vi "Peak Detection.vi"() -> ()   [LabVIEW 2015]
uses:
  <vilib>/Utility/file.llb/Read Delimited Spreadsheet (DBL).vi
  <userlib>/_OpenG.lib/array/array.llb/Sort 2D Array (DBL)__ogtk.vi
  <vilib>/Analysis/NI_AALPro.lvlib
  <vilib>/Analysis/NI_AAL_SigProc.lvlib
panel:
  out "Within 5 Peaks of each other?":bool[](array[boolean])
  out "Smoothed Data":dbl[](array[numeric])
  out "isDecreasing":bool[](array[boolean])
  out "isIncreasing":bool[](array[boolean])
  out "(2nd) Zero Crossing Amplitude and Index":dbl[][](array[numeric])
  out "(1st) Zero Crossing Amplitude and Index":dbl[][](array[numeric])
  out "Sorted 2D Array":sgl[][](array[numeric])
  in  "MinumumPeakHeightThresholdCounts":dbl format="%#_13g"
  out "?":cluster{dbl, dbl}[](graph)=[{0.0, 0.0}, {0.0, 0.0}, {366.0, 183.0}, {15.0, 190.5}, {11.0, 13.0}, {18.0, 14.5}, {9.0, 13.5}, {8.0, 8.5}, {0.0, 4.0}, {3.0, 1.5}, {11.0, 7.0}, {12.0, 11.5}, {16.0, 14.0}, {22.0, 19.0}, {16.0, 19.0}, {26.0, 21.0}, {17.0, 21.5}, {11.0, 14.0}, {1.0, 6.0}, {1.0, 1.0}, {0.0, 0.5}, {3.0, 1.5}, {4.0, 3.5}, {6.0, 5.0}, {16.0, 11.0}, {25.0, 20.5}, {53.0, 39.0}, {91.0, 72.0}, {204.0, 147.5}, {638.0, 421.0}, {2954.0, 1796.0}, {4799.0, 3876.5}, {6341.0, 5570.0}, {6306.0, 6323.5}, {6336.0, 6321.0}, {5904.0, 6120.0}, {5304.0, 5604.0}, {2436.0, 3870.0}, {107.0, 1271.5}, {17.0, 62.0}, {23.0, 20.0}, {82.0, 52.5}, {127.0, 104.5}, {93.0, 110.0}, {124.0, 108.5}, {109.0, 116.5}, {89.0, 99.0}, {58.0, 73.5}, {2.0, 30.0}, {3.0, 2.5}, {14.0, 8.5}, {25.0, 19.5}, {32.0, 28.5}, {37.0, 34.5}, {36.0, 36.5}, {29.0, 32.5}, {22.0, 25.5}, {9.0, 15.5}, {2.0, 5.5}, {1.0, 1.5}, {3.0, 2.0}, {5.0, 4.0}, {2.0, 3.5}, {2.0, 2.0}, {10.0, 6.0}, {14.0, 12.0}, {21.0, 17.5}, {22.0, 21.5}, {14.0, 18.0}, {24.0, 19.0}, {17.0, 20.5}, {10.0, 13.5}, {7.0, 8.5}, {10.0, 8.5}, {20.0, 15.0}, {36.0, 28.0}, {22.0, 29.0}, {56.0, 39.0}, {43.0, 49.5}, {64.0, 53.5}, {49.0, 56.5}, {23.0, 36.0}, {5.0, 14.0}, {11.0, 8.0}, {8.0, 9.5}, {17.0, 12.5}, {24.0, 20.5}, {20.0, 22.0}, {19.0, 19.5}, {28.0, 23.5}, {13.0, 20.5}, {14.0, 13.5}, {28.0, 21.0}, {61.0, 44.5}, {115.0, 88.0}, {186.0, 150.5}, {306.0, 246.0}, {305.0, 305.5}, {294.0, 299.5}, {338.0, 316.0}, {235.0, 286.5}, {236.0, 235.5}, {131.0, 183.5}, {51.0, 91.0}, {48.0, 49.5}, {81.0, 64.5}, {87.0, 84.0}, {112.0, 99.5}, {94.0, 103.0}, {103.0, 98.5}, {93.0, 98.0}, {71.0, 82.0}, {39.0, 55.0}, {24.0, 31.5}, {31.0, 27.5}, {51.0, 41.0}, {51.0, 51.0}, {62.0, 56.5}, {58.0, 60.0}, {53.0, 55.5}, {52.0, 52.5}, {62.0, 57.0}, {27.0, 44.5}, {5.0, 16.0}, {8.0, 6.5}, {4.0, 6.0}, {3.0, 3.5}, {3.0, 3.0}, {4.0, 3.5}, {15.0, 9.5}, {8.0, 11.5}, {15.0, 11.5}, {18.0, 16.5}, {15.0, 16.5}, {9.0, 12.0}, {4.0, 6.5}, {2.0, 3.0}, {2.0, 2.0}, {5.0, 3.5}, {7.0, 6.0}, {18.0, 12.5}, {14.0, 16.0}, {8.0, 11.0}, {13.0, 10.5}, {15.0, 14.0}, {40.0, 27.5}, {102.0, 71.0}, {227.0, 164.5}, {319.0, 273.0}, {462.0, 390.5}, {638.0, 550.0}, {643.0, 640.5}, {632.0, 637.5}, {620.0, 626.0}, {481.0, 550.5}, {361.0, 421.0}, {138.0, 249.5}, {121.0, 129.5}, {172.0, 146.5}, {275.0, 223.5}, {272.0, 273.5}, {352.0, 312.0}, {353.0, 352.5}, {267.0, 310.0}, {243.0, 255.0}, {167.0, 205.0}, {66.0, 116.5}, {56.0, 61.0}, {70.0, 63.0}, {93.0, 81.5}, {119.0, 106.0}, {129.0, 124.0}, {117.0, 123.0}, {92.0, 104.5}, {81.0, 86.5}, {48.0, 64.5}, {28.0, 38.0}, {22.0, 25.0}, {17.0, 19.5}, {25.0, 21.0}, {29.0, 27.0}, {34.0, 31.5}, {33.0, 33.5}, {31.0, 32.0}, {26.0, 28.5}, {16.0, 21.0}, {0.0, 8.0}, {0.0, 0.0}, {0.0, 0.0}, {0.0, 0.0}, {0.0, 0.0}, {0.0, 0.0}, {1.0, 0.5}, {2.0, 1.5}, {2.0, 2.0}, {2.0, 2.0}, {2.0, 2.0}, {0.0, 1.0}, {0.0, 0.0}, {3.0, 1.5}, {1.0, 2.0}, {1.0, 1.0}, {0.0, 0.5}, {2.0, 1.0}, {0.0, 1.0}, {0.0, 0.0}, {1.0, 0.5}, {2.0, 1.5}, {6.0, 4.0}, {21.0, 13.5}, {22.0, 21.5}, {33.0, 27.5}, {26.0, 29.5}, {35.0, 30.5}, {38.0, 36.5}, {49.0, 43.5}, {39.0, 44.0}, {23.0, 31.0}, {15.0, 19.0}, {8.0, 11.5}, {18.0, 13.0}, {26.0, 22.0}, {21.0, 23.5}, {37.0, 29.0}, {27.0, 32.0}, {32.0, 29.5}, {27.0, 29.5}, {24.0, 25.5}, {10.0, 17.0}, {6.0, 8.0}, {10.0, 8.0}, {11.0, 10.5}, {15.0, 13.0}, {14.0, 14.5}, {13.0, 13.5}, {10.0, 11.5}, {11.0, 10.5}, {5.0, 8.0}, {2.0, 3.5}, {4.0, 3.0}, {1.0, 2.5}, {5.0, 3.0}, {3.0, 4.0}, {4.0, 3.5}, {4.0, 4.0}, {3.0, 3.5}, {3.0, 3.0}, {2.0, 2.5}, {0.0, 1.0}, {0.0, 0.0}, {0.0, 0.0}, {1.0, 0.5}, {2.0, 1.5}, {1.0, 1.5}, {1.0, 1.0}, {0.0, 0.5}, {0.0, 0.0}, {0.0, 0.0}, {0.0, 0.0}, {0.0, 0.0}, {0.0, 0.0}, {0.0, 0.0}, {1.0, 0.5}, {0.0, 0.5}, {0.0, 0.0}, {0.0, 0.0}, {0.0, 0.0}, {1.0, 0.5}, {0.0, 0.5}, {0.0, 0.0}, {3.0, 1.5}, {2.0, 2.5}, {8.0, 5.0}, {11.0, 9.5}, {9.0, 10.0}, {21.0, 15.0}, {21.0, 21.0}, {11.0, 16.0}, {8.0, 9.5}, {4.0, 6.0}, {2.0, 3.0}, {4.0, 3.0}, {9.0, 6.5}, {12.0, 10.5}, {8.0, 10.0}, {9.0, 8.5}, {11.0, 10.0}, {12.0, 11.5}, {4.0, 8.0}, {5.0, 4.5}, {0.0, 2.5}, {3.0, 1.5}, {7.0, 5.0}, {6.0, 6.5}, {6.0, 6.0}, {4.0, 5.0}, {6.0, 5.0}, {2.0, 4.0}, {1.0, 1.5}, {0.0, 0.5}, {0.0, 0.0}, {1.0, 0.5}, {2.0, 1.5}, {1.0, 1.5}, {1.0, 1.0}, {2.0, 1.5}, {5.0, 3.5}, {1.0, 3.0}, {0.0, 0.5}, {0.0, 0.0}, {0.0, 0.0}, {0.0, 0.0}, {0.0, 0.0}, {0.0, 0.0}, {1.0, 0.5}, {0.0, 0.5}, {0.0, 0.0}, {0.0, 0.0}, {0.0, 0.0}, {0.0, 0.0}, {1.0, 0.5}, {0.0, 0.5}, {0.0, 0.0}, {0.0, 0.0}, {1.0, 0.5}, {0.0, 0.5}, {0.0, 0.0}, {0.0, 0.0}, {0.0, 0.0}, {0.0, 0.0}, {0.0, 0.0}, {0.0, 0.0}, {0.0, 0.0}, {1.0, 0.5}, {2.0, 1.5}, {2.0, 2.0}, {3.0, 2.5}, {2.0, 2.5}, {4.0, 3.0}, {4.0, 4.0}, {3.0, 3.5}, {1.0, 2.0}, {1.0, 1.0}, {3.0, 2.0}, {1.0, 2.0}, {0.0, 0.5}, {2.0, 1.0}, {2.0, 2.0}, {0.0, 1.0}, {1.0, 0.5}, {1.0, 1.0}, {0.0, 0.5}, {1.0, 0.5}, {1.0, 1.0}, {0.0, 0.5}, {0.0, 0.0}, {0.0, 0.0}, {0.0, 0.0}, {1.0, 0.5}, {1.0, 1.0}, {0.0, 0.5}, {0.0, 0.0}, {0.0, 0.0}, {1.0, 0.5}, {0.0, 0.5}, {0.0, 0.0}, {0.0, 0.0}, {2.0, 1.0}, {0.0, 1.0}, {0.0, 0.0}]
  in  "MinimumPeakHeightThresholdFunction":dbl format="%#_13g"
  in  "MinimumPeakWidth":dbl format="%#_13g"
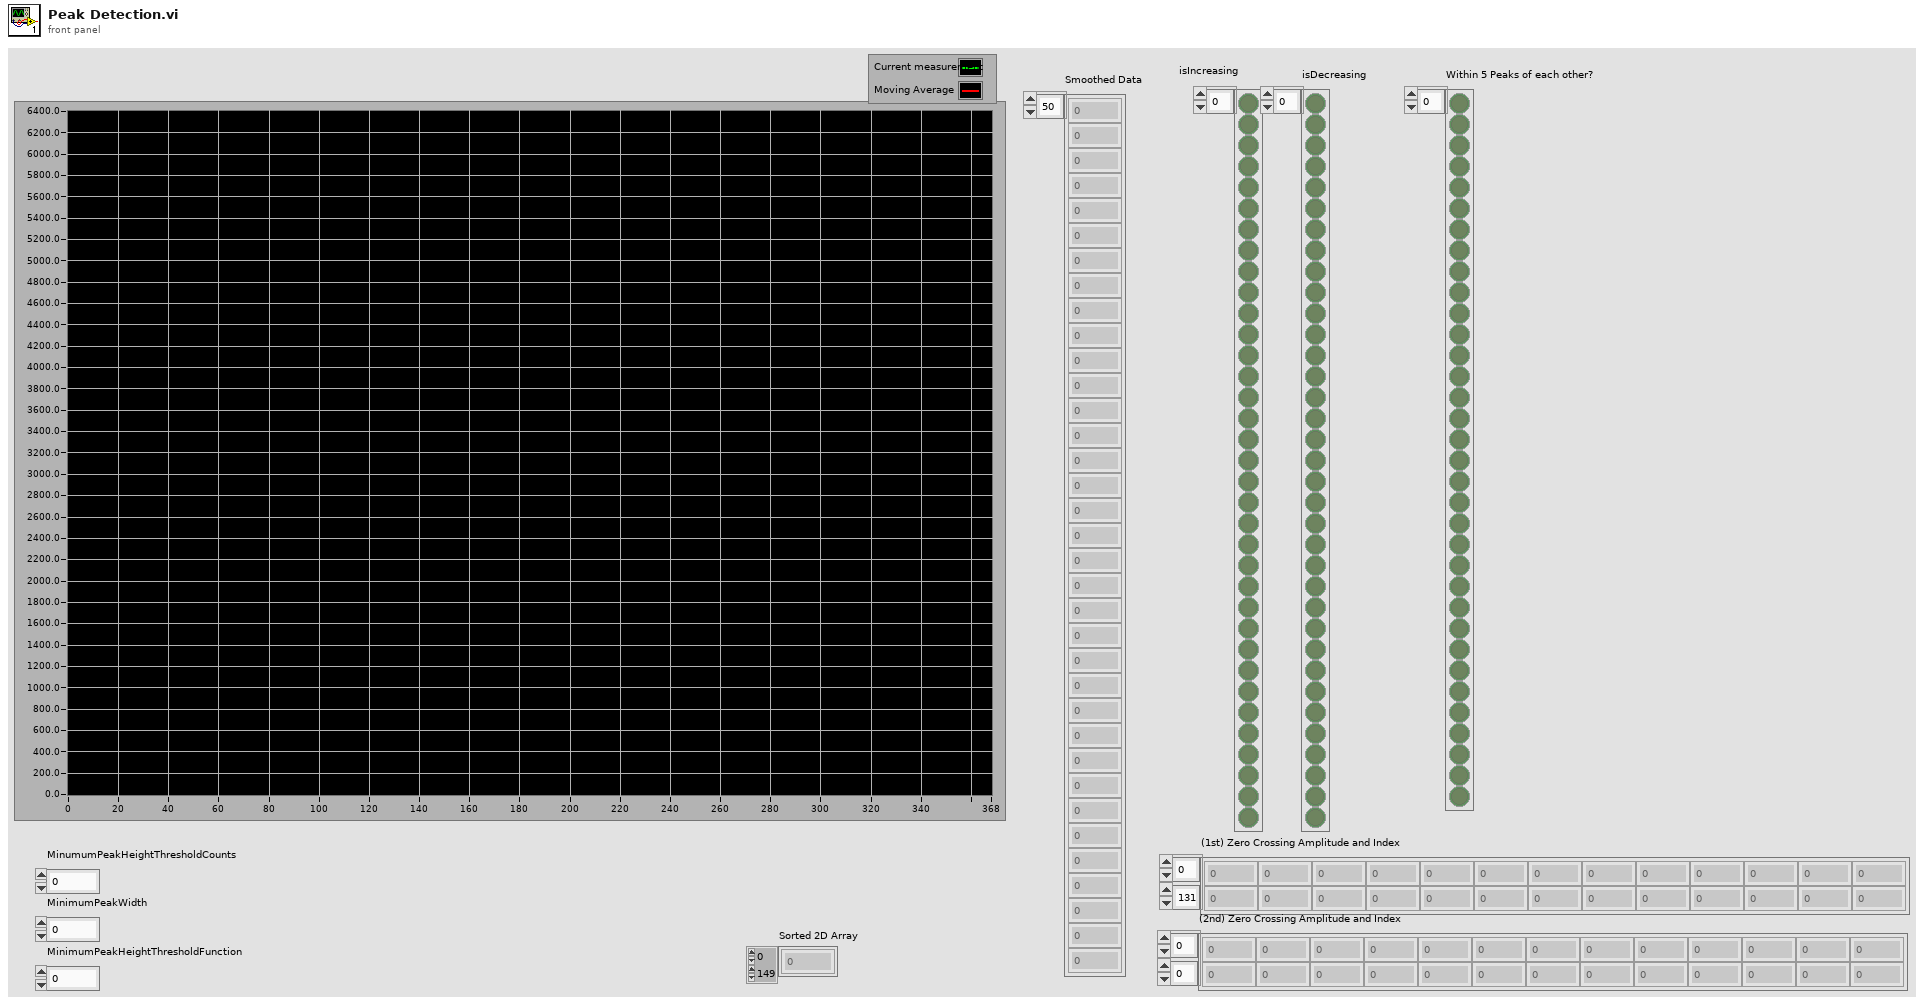
[diagram p1: front panel]
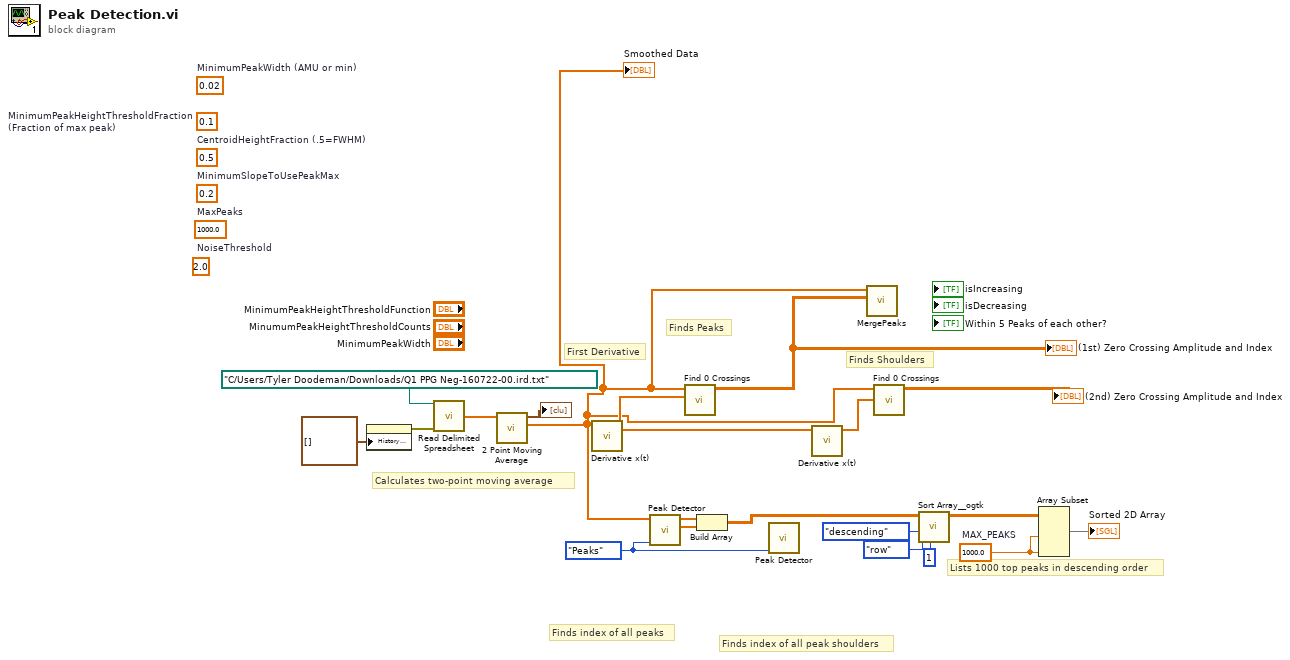
[diagram p0: block diagram]
diagram:
  (unwired) 1000.0  # MaxPeaks
  (unwired) 2.0  # NoiseThreshold
  (unwired) 0.2  # MinimumSlopeToUsePeakMax
  (unwired) 0.5  # CentroidHeightFraction (.5=FWHM)
  (unwired) 0.1  # MinimumPeakHeightThresholdFraction (Fraction of max peak)
  (unwired) 0.02  # MinimumPeakWidth (AMU or min)
  w10 = 1000.0  # MAX_PEAKS
  w19 = enum32{"Peaks", "Valleys"}."Peaks" ("peaks/valleys")
  # "Finds Shoulders"
  # "Finds Peaks"
  # "First Derivative"
  # "Lists 1000 top peaks in descending order"
  # "Finds index of all peak shoulders"
  # "Finds index of all peaks"
  # "Calculates two-point moving average"
  n1 = property class="WFChart (strict)"("History Data"=cluster{dbl, dbl}[] []) -> (error out=w6:errorcluster)  [unwired: 2 in, 1 out]
  n2 = call-poly <vilib>:"Read Delimited Spreadsheet.vi"("file path (dialog if empty)"=path "C:/Users/Tyler Doodeman/Downloads/Q1 PPG Neg-160722-00.ird.txt", "error in (no error)"=w6) -> ("first row"=w7:dbl[])  [unwired: 8 in, 5 out]
  n3 = call "2 Point Moving Average.vi"("Peak Data"=w7) -> ("Smoothed Data"=w1:dbl[], "Orig VS Smoothed"=→"?":cluster{dbl, dbl}[])  [unwired: 9 in]
  "Smoothed Data" <- w1
  n4 = call <vilib>:"Derivative x(t).vi"("X"=w1) -> ("dX/dt"=w5:dbl[])  [unwired: 9 in, 1 out]
  n5 = call <vilib>:"Peak Detector.vi"("peaks/valleys"=w19, "X"=w1) -> ("Amplitudes"=w17:dbl[], "Locations"=w18:dbl[])  [unwired: 5 in, 3 out]
  n6 = call "Find 0 Crossings.vi"("dX/dt"=w5, "Smoothed Data"=w1) -> ("Array"=w2:dbl[][])  [unwired: 9 in]
  "(1st) Zero Crossing Amplitude and Index" <- w2
  n7 = Build Array(w18, w17) -> (w13:dbl[][])
  n8 = call <vilib>:"Peak Detector.vi"("peaks/valleys"=w19) -> ()  [unwired: 6 in, 5 out]
  n9 = call <vilib>:"Derivative x(t).vi"("X"=w5) -> ("dX/dt"=w4:dbl[])  [unwired: 9 in, 1 out]
  n10 = call "MergePeaks.vi"("Array"=w2, "Smoothed Data"=w1) -> ()  [unwired: 10 in]
  n11 = call "Find 0 Crossings.vi"("dX/dt"=w4, "Smoothed Data"=w1) -> ("Array"=→"(2nd) Zero Crossing Amplitude and Index":dbl[][])  [unwired: 9 in]
  n12 = call-poly <userlib>:"Sort Array__ogtk.vi"("Column/Row to Sort By"=u32 1, "Sort By in"=enum16{"row", "column"}."row", "Order"=enum16{"ascending", "descending"}."descending", "Array in"=w13) -> ("Sorted Array out"=w12:dbl[][])  [unwired: 4 in, 3 out]
  n13 = Array Subset(array=w12, length (row)=w10, length (col)=w10) -> (→"Sorted 2D Array":dbl[][])  [unwired: 2 in]
